vi "CRYStimulus.vi"(0 "Setup in":T2={"No.VI"=0, "Category"="", "StepName"="", "Seq setup flattened"="", "Comment"="", "Steps config."=[], "Jump config"=[], "Start"=0.0, "Increment"=0.0, "Name"="Pa", "Unit"="Pa", "Y data"=1, "Y prefix"="", "Y dB ref"=1.0, "Y unit"="", "Repeat State Array"=[]} {"Repeat State Array"."Start" format="%#_5g"; "Y dB ref" format="%.1f"; "Y data" items=["dB", "Lin"]; "Start" format="%#_5g"}, 5 "Data in":T10 {"Z data" items=["dB", "Lin"]; "X data" items=["dB", "Lin"]; "Y data" items=["dB", "Lin"]; "Z dB ref" format="%.1f"; "Z axis" items=["Log", "Lin"]; "X dB ref" format="%.1f"; "X axis" items=["Log", "Lin"]; "Y axis" items=["Log", "Lin"]; "Y dB ref" format="%.1f"; "Curve"."z" format="%.2f"; "Curve"."y" format="%.2f"; "Curve"."x" format="%.2f"}, 7 "Results in":T8 {"Margin" format="%.2f"}, 9 "Seq Setup in":string, 11 "Step name":string, 12 "Hardware in":string, 13 "Calibration in":string) -> (3 "Types Out":string[](array[string]), 4 "Inserted Names Out":string[](array[string]), 6 "Data out":T10 {"Z data" items=["dB", "Lin"]; "X data" items=["dB", "Lin"]; "Y data" items=["dB", "Lin"]; "Z dB ref" format="%.1f"; "Z axis" items=["Log", "Lin"]; "X dB ref" format="%.1f"; "X axis" items=["Log", "Lin"]; "Y axis" items=["Log", "Lin"]; "Y dB ref" format="%.1f"; "Curve"."z" format="%.2f"; "Curve"."y" format="%.2f"; "Curve"."x" format="%.2f"}, 8 "Results out":T8 {"Margin" format="%.2f"}, 10 "Wave out":T1[](array[typedef]) {"Y dB ref" format="%.1f"; "Y axis" items=["Log", "Lin"]; "Y data" items=["dB", "Lin"]; "X data" items=["dB", "Lin"]})   [LabVIEW 2013]
uses:
  Typedef Control/CRYData Cluster Array.ctl
  Typedef Control/CRYData Cluster.ctl
  Typedef Control/CRYResult Cluster Array.ctl
  Typedef Control/CRYResult Cluster.ctl
  Typedef Control/CRYWaveform Cluster.ctl
  Typedef Control/CRYCalibration 2DCluster.ctl
  Typedef Control/CRYCalibration Cluster.ctl
  Typedef Control/CRYStep.ctl
  Typedef Control/CRYStimulus Test Infor Cluster.ctl
  CRYMainGlobal.vi
  Task Sequence/CRYProject Run Control Global.vi
  Hardware/SubVI/CRY6175APT_Win32.dll
panel:
  out "Unit":u16
  out "Stop Amplitude":dbl
  in  "Start Amplitude":dbl
  in  "Frequency":dbl
  out "Steps":u32
  out "Resolution":u16
  in  "Stop Frequency":dbl
  in  "Start Frequency":dbl
  in  "Level Out":dbl
  in  "Sampling Rate":dbl
  in  "Sweep Time":dbl
  in  "Channel Out":i32=5
  out "use level":bool
  out "EQ Amplitude Rate":dbl
  out "Y dB ref":dbl
  in  "Waveform Cluster":T1={"Waveform"={"X0"=0.0, "dX"=0.0, "Y"=[]}, "X data"=1, "Y data"=0, "Y axis"=0, "X unit"="s", "Y unit"="", "Y dB ref"=1.0, "display Y"=TRUE, "display X"=FALSE, "Overload?"=FALSE, "Test Info"="", "Step No."=0, "Name"="", "protected"=FALSE, "Sqc history"=[], "Signal Channel ID"=0, "Plot Settings"={"Color"=0, "Interpolation"=0, "Point Style"=0, "Line Style"=0, "Point Color"=0, "Line Width"=0, "Bar Plot Style"=0, "Fill To"=0}, "AutoProtect"=FALSE} {"Y dB ref" format="%.1f"; "Y axis" items=["Log", "Lin"]; "Y data" items=["dB", "Lin"]; "X data" items=["dB", "Lin"]}
  out "EQ Curve":T3={"Name"="", "Curve"=[], "X data"=1, "Y data"=1, "Z data"=1, "X axis"=0, "Y axis"=1, "Z axis"=1, "X unit"="Hz", "Y unit"="", "Z unit"="deg.", "X dB ref"=1.0, "Y dB ref"=1.0, "Z dB ref"=1.0, "single val"=FALSE, "protected"=FALSE, "display X"=TRUE, "display Y"=TRUE, "display Z"=TRUE, "Test Info"="", "Step No."=0, "Plot Settings"={"Color"=0, "Interpolation"=0, "Point Style"=0, "Line Style"=0, "Point Color"=0, "Line Width"=0, "Bar Plot Style"=0, "Fill To"=0}, "AutoProtect"=FALSE} {"Z data" items=["dB", "Lin"]; "X data" items=["dB", "Lin"]; "Y data" items=["dB", "Lin"]; "Z dB ref" format="%.1f"; "Z axis" items=["Log", "Lin"]; "X dB ref" format="%.1f"; "X axis" items=["Log", "Lin"]; "Y axis" items=["Log", "Lin"]; "Y dB ref" format="%.1f"; "Curve"."z" format="%.2f"; "Curve"."y" format="%.2f"; "Curve"."x" format="%.2f"}
  out "Calibration All Cluster":T4={"Calibration"={"Calibration Step Name"="", "Device"="", "Correction Curve Name"="", "Equalization Curve Name"="", "Sensitivity Curve Name"="", "Corr Folder and File"="", "EQ Folder and File"="", "Sens Folder and File"="", "Corr Step size"=0, "EQ Step size"=0, "Input"=FALSE, "Last Cal Date (sec)"=timestamp(0 s since 1904-01-01), "Cha Name"="", "Corr Curve Found"=FALSE, "EQ Curve Found"=FALSE, "Sens Curve Found"=FALSE, "Signal Type"="", "Calibrated Device"="", "Hz"=0}, "Corr Curve"={"Name"="", "Curve"=[], "X data"=1, "Y data"=1, "Z data"=1, "X axis"=0, "Y axis"=1, "Z axis"=1, "X unit"="", "Y unit"="", "Z unit"="deg.", "X dB ref"=1.0, "Y dB ref"=1.0, "Z dB ref"=1.0, "single val"=FALSE, "protected"=FALSE, "display X"=FALSE, "display Y"=TRUE, "display Z"=TRUE, "Test Info"="", "Step No."=0, "Plot Settings"={"Color"=0, "Interpolation"=0, "Point Style"=0, "Line Style"=0, "Point Color"=0, "Line Width"=0, "Bar Plot Style"=0, "Fill To"=0}, "AutoProtect"=FALSE}, "EQ Curve"={"Name"="", "Curve"=[], "X data"=1, "Y data"=1, "Z data"=1, "X axis"=0, "Y axis"=1, "Z axis"=1, "X unit"="Hz", "Y unit"="", "Z unit"="deg.", "X dB ref"=1.0, "Y dB ref"=1.0, "Z dB ref"=1.0, "single val"=FALSE, "protected"=FALSE, "display X"=TRUE, "display Y"=TRUE, "display Z"=TRUE, "Test Info"="", "Step No."=0, "Plot Settings"={"Color"=0, "Interpolation"=0, "Point Style"=0, "Line Style"=0, "Point Color"=0, "Line Width"=0, "Bar Plot Style"=0, "Fill To"=0}, "AutoProtect"=FALSE}, "Sens Curve"={"Name"="", "Curve"=[], "X data"=1, "Y data"=1, "Z data"=1, "X axis"=0, "Y axis"=1, "Z axis"=1, "X unit"="Hz", "Y unit"="", "Z unit"="deg.", "X dB ref"=1.0, "Y dB ref"=1.0, "Z dB ref"=1.0, "single val"=FALSE, "protected"=FALSE, "display X"=TRUE, "display Y"=TRUE, "display Z"=TRUE, "Test Info"="", "Step No."=0, "Plot Settings"={"Color"=0, "Interpolation"=0, "Point Style"=0, "Line Style"=0, "Point Color"=0, "Line Width"=0, "Bar Plot Style"=0, "Fill To"=0}, "AutoProtect"=FALSE}} {"Sens Curve"."Z data" items=["dB", "Lin"]; "Sens Curve"."X data" items=["dB", "Lin"]; "Sens Curve"."Y data" items=["dB", "Lin"]; "Sens Curve"."Z dB ref" format="%.1f"; "Sens Curve"."Z axis" items=["Log", "Lin"]; "Sens Curve"."X dB ref" format="%.1f"; "Sens Curve"."X axis" items=["Log", "Lin"]; "Sens Curve"."Y axis" items=["Log", "Lin"]; "Sens Curve"."Y dB ref" format="%.1f"; "Sens Curve"."Curve"."z" format="%.2f"; "Sens Curve"."Curve"."y" format="%.2f"; "Sens Curve"."Curve"."x" format="%.2f"; "EQ Curve"."Z data" items=["dB", "Lin"]; "EQ Curve"."X data" items=["dB", "Lin"]; "EQ Curve"."Y data" items=["dB", "Lin"]; "EQ Curve"."Z dB ref" format="%.1f"; "EQ Curve"."Z axis" items=["Log", "Lin"]; "EQ Curve"."X dB ref" format="%.1f"; "EQ Curve"."X axis" items=["Log", "Lin"]; "EQ Curve"."Y axis" items=["Log", "Lin"]; "EQ Curve"."Y dB ref" format="%.1f"; "EQ Curve"."Curve"."z" format="%.2f"; "EQ Curve"."Curve"."y" format="%.2f"; "EQ Curve"."Curve"."x" format="%.2f"; "Corr Curve"."Z data" items=["dB", "Lin"]; "Corr Curve"."X data" items=["dB", "Lin"]; "Corr Curve"."Y data" items=["dB", "Lin"]; "Corr Curve"."Z dB ref" format="%.1f"; "Corr Curve"."Z axis" items=["Log", "Lin"]; "Corr Curve"."X dB ref" format="%.1f"; "Corr Curve"."X axis" items=["Log", "Lin"]; "Corr Curve"."Y axis" items=["Log", "Lin"]; "Corr Curve"."Y dB ref" format="%.1f"; "Corr Curve"."Curve"."z" format="%.2f"; "Corr Curve"."Curve"."y" format="%.2f"; "Corr Curve"."Curve"."x" format="%.2f"; "Calibration"."EQ Step size" items=["R10", "R20", "R40", "R80", "User"]; "Calibration"."Corr Step size" items=["R10", "R20", "R40", "R80", "User"]}
  out "Analysis Value":dbl[](array[numeric])
  out "TSR params":T6 {"Sweep Time" format="%.2f"; "Amplit" format="%.2f"; "FStop" format="%.2f"; "FStart" format="%.2f"; "FSamp" format="%.2f"; "Tsamp" format="%.2f"; "NHarm" format="%.2f"; "MStart" format="%.2f"; "MStop" format="%.2f"; "NOffset" format="%.2f"}
  out "FAPS":T7(array[cluster]) {"cycles" format="%.2f"; "ampl" format="%.2f"; "freq" format="%.2f"}
  in  "Channel In":i32
  in  "wav path":path
  in  "max level":dbl format="%.2f"
  in  "Eq":cluster{"Hz":sgl, "dB":sgl, "Deg":sgl}[](array[cluster]) {"Deg" format="%.1f"; "dB" format="%.1f"}
  out "EQ Step size":u16(ring)=4 items=["R10", "R20", "R40", "R80", "User"]
  out "EQ Steps":i32=19
  in  "sine waves":cluster{"freq":dbl, "ampl":dbl, "cycles":dbl}[](array[cluster]) {"cycles" format="%.2f"; "ampl" format="%.2f"; "freq" format="%.2f"}
  in  "sweep type":i32
  out "Y unit":string
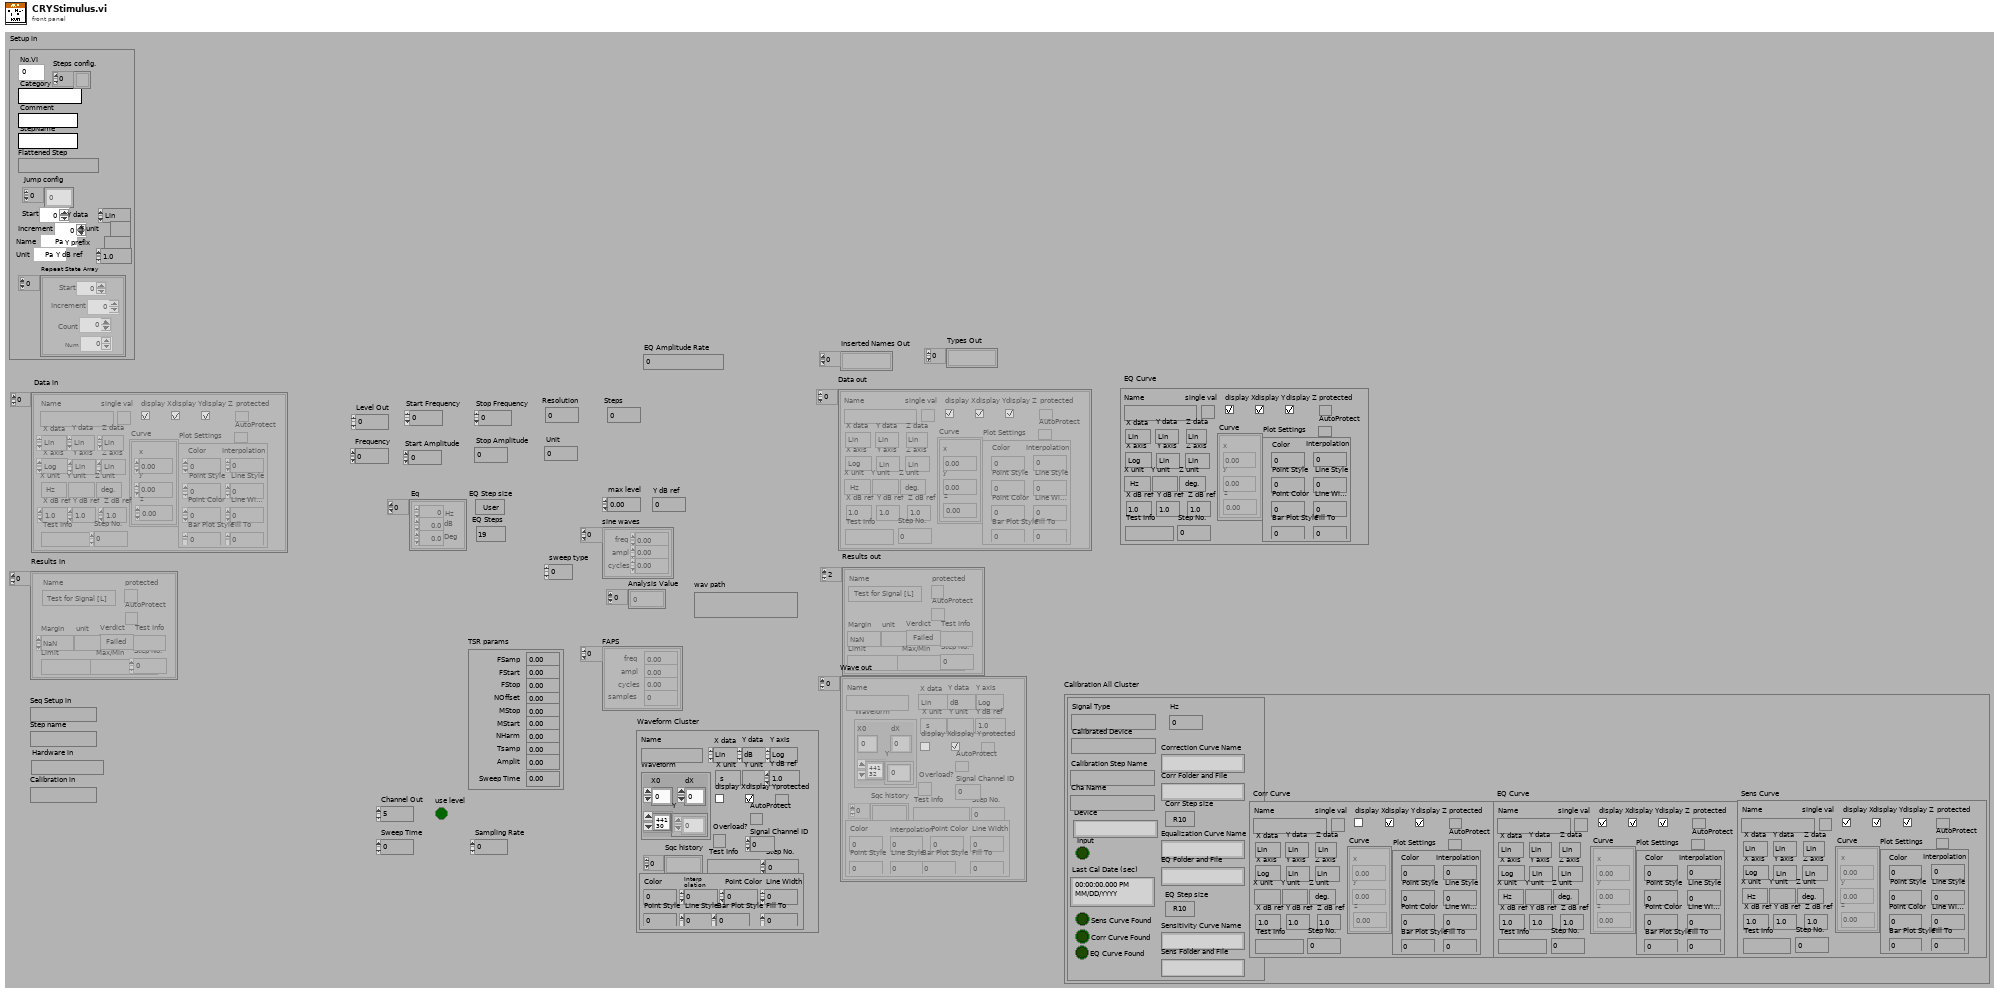
[diagram p1: front panel]
types:
  T1 = typedef "CRYWaveform Cluster.ctl" = cluster{"Waveform":cluster{"X0":dbl, "dX":dbl, "Y":sgl[]}, "X data":u16, "Y data":u16, "Y axis":u16, "X unit":string, "Y unit":string, "Y dB ref":dbl, "display Y":bool, "display X":bool, "Overload?":bool, "Test Info":string, "Step No.":i32, "Name":string, "protected":bool, "Sqc history":string[], "Signal Channel ID":i32, "Plot Settings":cluster{"Color":u32, "Interpolation":u8, "Point Style":u8, "Line Style":u8, "Point Color":u32, "Line Width":u8, "Bar Plot Style":u8, "Fill To":i16}, "AutoProtect":bool}
  T2 = typedef "CRYStep.ctl" = cluster{"No.VI":i32, "Category":string, "StepName":string, "Seq setup flattened":string, "Comment":string, "Steps config.":bool[], "Jump config":i32[], "Start":dbl, "Increment":dbl, "Name":string, "Unit":string, "Y data":u16, "Y prefix":string, "Y dB ref":dbl, "Y unit":string, "Repeat State Array":cluster{"Start":dbl, "Increment":dbl, "Count":i32, "Num":i32}[]}
  T3 = typedef "CRYData Cluster.ctl" = cluster{"Name":string, "Curve":cluster{"x":dbl, "y":dbl, "z":dbl}[], "X data":u16, "Y data":u16, "Z data":u16, "X axis":u16, "Y axis":u16, "Z axis":u16, "X unit":string, "Y unit":string, "Z unit":string, "X dB ref":dbl, "Y dB ref":dbl, "Z dB ref":dbl, "single val":bool, "protected":bool, "display X":bool, "display Y":bool, "display Z":bool, "Test Info":string, "Step No.":i32, "Plot Settings":cluster{"Color":u32, "Interpolation":u8, "Point Style":u8, "Line Style":u8, "Point Color":u32, "Line Width":u8, "Bar Plot Style":u8, "Fill To":i16}, "AutoProtect":bool}
  T4 = typedef "CRYCalibration 2DCluster.ctl" = cluster{"Calibration":T5, "Corr Curve":T3, "EQ Curve":T3, "Sens Curve":T3}
  T5 = typedef "CRYCalibration Cluster.ctl" = cluster{"Calibration Step Name":string, "Device":string, "Correction Curve Name":string, "Equalization Curve Name":string, "Sensitivity Curve Name":string, "Corr Folder and File":string, "EQ Folder and File":string, "Sens Folder and File":string, "Corr Step size":u16, "EQ Step size":u16, "Input":bool, "Last Cal Date (sec)":timestamp, "Cha Name":string, "Corr Curve Found":bool, "EQ Curve Found":bool, "Sens Curve Found":bool, "Signal Type":string, "Calibrated Device":string, "Hz":u32}
  T6 = cluster{"FSamp":dbl, "FStart":dbl, "FStop":dbl, "NOffset":dbl, "MStop":dbl, "MStart":dbl, "NHarm":dbl, "Tsamp":dbl, "Amplit":dbl, "Sweep Time":dbl}
  T7 = cluster{"freq":dbl, "ampl":dbl, "cycles":dbl, "samples":i32}[]
  T8 = typedef "CRYResult Cluster Array.ctl" = T9[]
  T9 = typedef "CRYResult Cluster.ctl" = cluster{"Name":string, "Margin":dbl, "unit":string, "Verdict":bool, "Limit":string, "Max/Min":string, "protected":bool, "Step No.":i32, "Test Info":string, "AutoProtect":bool}
  T10 = typedef "CRYData Cluster Array.ctl" = T3[]
  T11 = enum16{"OK", "Yes", "YesNo", "YesNoCancel", "ReplaceAppend"}
  T12 = cluster{"FSamp":dbl, "FStart":dbl, "FStop":dbl, "NOffset":dbl, "MStop":dbl, "MStart":dbl, "NHarm":dbl, "Tsamp":dbl, "Amplit":dbl, "Amplit 2":dbl}
  T13 = cluster{"Start":dbl, "Increment":dbl, "Count":i32, "Num":i32}[]
  T14 = typedef "CRYStimulus Cluster.ctl" = cluster{"StimulusType":string, "UseMLValArray":u16[], "ML_axisArray":u16[], "MLValLevelNameArray":string[], "Level(U)Array":dbl[], "Start(Stop)FreqArray":dbl[], "Start(Stop)AmpArray":dbl[], "StepResolutionArray":u16[], "Unit_Array":u16[], "DegValArray":dbl[], "DegUnitArray":string[], "Steps1":i32, "Cycle/step1(#)":u32, "Time/step1(s)":dbl, "Transition1":dbl, "SweepRate2":dbl, "Freq3(Hz)":dbl, "Steps3(#)":dbl, "Cycles3(#)":u32, "StepSize3":dbl, "wave time":string, "RMS_Value4":dbl, "Peak_Value4":dbl, "WavePath4":string, "RMS_unit4":string, "Peak_unit4":string, "wave Info":string, "dc_ctrl5_1":u16, "dc_ctrl5_2":u16, "dc_polar5":u16, "Max.Current":u16, "Steps5(#)":u32, "Time/Step5":dbl, "Level5":dbl, "StepsSize5Val":dbl, "StepSize5Unit":string, "SweepType":u16, "Fixed/Ratio6":u16, "Transition6":dbl, "Steps6(#)":dbl, "Cycle/Steps6(#)":u32, "Time/Steps6(s)":dbl, "Freq6(Hz)":dbl, "Difference6(Hz)":dbl, "Ratio6":string, "NoiseType7":u16, "Duration7(s)":dbl, "MinFreq7(Hz)":dbl, "MaxFreq7(Hz)":dbl, "MinFreq8(Hz)":dbl, "MaxFreq8(Hz)":dbl, "FreqRounding8":bool, "Duration8(s)":dbl, "Tones8":dbl, "RoundingVal8":dbl, "ApplyEQ":bool, "Duration(s)":dbl, "CustomStimulusName ":string, "Flatten Element Array":string[], "sine waves":cluster{"freq":dbl, "ampl":dbl, "cycles":dbl}[], "Channel Out":i32, "RatioVal6":dbl, "TabCtrl6":enum32{"Master Tone", "Slave Tone"}, "Signal Type Name":string, "Help":string, "Channel Sel":u16, "V on DUT":bool, "Output Imp":dbl, "Nominal Imp":dbl}
  T15 = typedef "CRYStimulus Parameter.ctl" = cluster{"Name":string, "Level Out":dbl, "Start Freq":dbl, "Stop Freq":dbl, "Steps":u32, "Cycles":u32, "Sweep type":i32, "Freq":dbl, "Start ampl":dbl, "Stop ampl":dbl, "sine waves":cluster{"freq":dbl, "ampl":dbl, "cycles":dbl}[], "wav path":string, "Sweep time":dbl, "Resolution":u16, "Tone type6":u16, "fix/ratio6":u16, "Ratio6":u16, "Difference6":u32, "RatioFreq6":u32}
  T16 = typedef "CRYfstepsw.ctl" = cluster{"Level(U)":dbl, "Start Freq(Hz)":dbl, "Stop Freq(Hz)":dbl, "ML val level name":string, "Use ML Val level?":bool, "ML axis":u8, "Steps (#)":i32, "Cycles/step(#)":u32, "Time/step (s)":dbl, "Step Resolution":u16, "unit":u16, "Start Freq Name":string, "Stop Freq Name":string, "Start Freq Axis":u8, "Stop Freq Axis":u8, "Start Freq Flag":string, "Stop Freq Flag":string, "Output Imp":dbl, "Nominal Imp":dbl, "V on DUT":bool}
  T17 = typedef "CRYflogsw.ctl" = cluster{"Level(U)":dbl, "Start Freq(Hz)":dbl, "Stop Freq(Hz)":dbl, "Sweep Rate(s/dec)":dbl, "Use ML Val level?":bool, "ML val level name":string, "ML axis":u8, "TSR params":cluster{"FSamp":dbl, "FStart":dbl, "FStop":dbl, "NOffset":dbl, "MStop":dbl, "MStart":dbl, "NHarm":dbl, "Tsamp":dbl, "Amplit":dbl}, "unit":u16, "Start Freq Name":string, "Stop Freq Name":string, "Start Freq Axis":u8, "Stop Freq Axis":u8, "Start Freq Flag":string, "Stop Freq Flag":string, "Output Imp":dbl, "Nominal Imp":dbl, "V on DUT":bool}
  T18 = typedef "CRYampsw.ctl" = cluster{"Freq(Hz)":dbl, "Steps (#)":i32, "Cycles(#)":u32, "Use ML Val freq?":bool, "ML val freq name":string, "ML axis":u8, "Start Ampl(U)":dbl, "Stop Ampl(U)":dbl, "unit":u16}
  T19 = typedef "CRYwavefile.ctl" = cluster{"Level(U)":dbl, "Wave Path":string, "ML axis":u8, "ML val level name":string, "Use ML Val level?":bool, "wave info":string, "wave time":string, "Peak value4":dbl, "RMS value4":dbl, "wave channel":u16, "unit":u16, "Output Imp":dbl, "Nominal Imp":dbl, "V on DUT":bool}
  T20 = typedef "CRYdcconn.ctl" = cluster{"dc ctrl":u16, "dcmax I":u16, "dc polar":u16, "dc ctrl":u16, "Steps (#)":i32, "Time/step (s)":dbl, "Start Ampl(U)":dbl, "Stop Ampl(U)":dbl, "Level(U)":dbl, "Step Size":dbl}
  T21 = typedef "CRYtwotone.ctl" = cluster{"Steps (#)":i32, "Tone Type":u8, "Freq2(Hz)":dbl, "Time/step (s)":dbl, "Cycles/step (#)":u32, "ML val level name":string, "Use ML Val level?":bool, "Level(U) 2":dbl, "Diff Freq(Hz)":dbl, "ML axis 2":u8, "Diff/Ratio":u8, "Level(U)":dbl, "Stop Freq(Hz)":dbl, "Ratio Val":dbl, "ML val level name 2":string, "Use ML Val level? 2":bool, "ML axis":u8, "Start Freq(Hz)":dbl, "Step Resolution":u16, "Ratio":u16, "TabCtrl6":enum32{"Master Tone", "Slave Tone"}, "unit 1":u16, "unit 2":u16, "Start Freq Name":string, "Stop Freq Name":string, "Start Freq Axis":u8, "Stop Freq Axis":u8, "Start Freq Flag":string, "Stop Freq Flag":string}
  T22 = typedef "CRYmltitone.ctl" = cluster{"Level(U)":dbl, "Min Freq(Hz)":dbl, "Max Freq(Hz)":dbl, "Duration(s)":dbl, "Freq Rounding":bool, "Rounding Val":dbl, "Profile":i32, "ML axis 2":u8, "ML val level name":string, "Use ML Val level?":bool, "ML axis":u8, "Step Resolution":u16, "unit":u16, "Start Freq Name":string, "Stop Freq Name":string, "Start Freq Axis":u8, "Stop Freq Axis":u8, "Start Freq Flag":string, "Stop Freq Flag":string, "Output Imp":dbl, "Nominal Imp":dbl, "V on DUT":bool}
  T23 = typedef "CRYnoise.ctl" = cluster{"Noise Type":u8, "Min Freq(Hz)":dbl, "Max Freq(Hz)":dbl, "Level(U)":dbl, "Duration(s)":dbl, "ML val level name":string, "Use ML Val level?":bool, "ML axis":u8, "unit":u16, "Start Freq Name":string, "Stop Freq Name":string, "Start Freq Axis":u8, "Stop Freq Axis":u8, "Start Freq Flag":string, "Stop Freq Flag":string, "Output Imp":dbl, "Nominal Imp":dbl, "V on DUT":bool}
  T24 = cluster{"fstepsw":T16, "flogsw":T17, "ampsw":T18, "wavefile":T19, "dcconn":T20, "twotone":T21, "mltitone":T22, "noise":T23, "sqwvsw":cluster{"Level(U)":dbl, "Duty Cycle":dbl, "ML val level name":string, "ML axis":u8, "Start Freq(Hz)":u32, "Stop Freq(Hz)":u32, "Use ML Val level?":bool, "Steps (#)":u32, "Cycles/step (#)":u32, "Time/step (s)":dbl, "Step Resolution":u16}, "tnbrst":cluster{"Level(U)":dbl, "ML val level name":string, "ML axis":u8, "Start Freq(Hz)":u32, "Use ML Val level?":bool, "Cycles/step (#)":u32, "Duration(s)":dbl}}
  T25 = typedef "CRYHardware Channel Info.ctl" = cluster{"ID":i32, "Name":string, "Digital":bool, "Input":bool, "Device Name":string, "Hardware Ch ID":u8, "Vmax (V)":dbl, "Latency (samples)":dbl, "Sampling Rate (Hz)":u32, "Bit Depth":u32, "Anti-aliasing Factor (%fs)":sgl, "DAQmx Channel":tag, "term config":i32, "Coupling":i32, "IEPE en":bool, "ASIOChannel Name":string, "Audio Driver":u16, "ASIOChannel Index":u8}
  T26 = cluster{"sweep type":i32, "Sampling Rate":dbl, "Frequency":dbl, "Start Amplitude":dbl, "Level Out":dbl}
  T27 = cluster{"Unit":u16, "max level":dbl, "Y dB ref":dbl}
  T28 = cluster{"Start Frequency":dbl, "Stop Frequency":dbl, "Steps":u32, "Sweep Time":dbl, "Level Out":dbl, "Level Out":dbl, "Unit":u16, "max level":dbl, "Y dB ref":dbl}
  T29 = typedef "CRYStimulus Test Infor Cluster.ctl" = cluster{"Stimulus Type":string, "Signal Type":string, "In/Out":bool, "FAPS":cluster{"freq":dbl, "ampl":dbl, "cycles":dbl, "samples":i32}[], "Sampling Rate":dbl, "Samples":i32, "Analysis Param":string, "Resolution":u16, "Steps":u32, "Analysis Value":dbl[], "Diff Freq":dbl, "FStart":dbl, "FStop":dbl, "Calibration Param":string, "Anti Alias":dbl, "Level Out1":dbl, "Level Out2":dbl, "EQ":bool}
  T30 = typedef "CRYWaveform Cluster Array.ctl" = T1[]
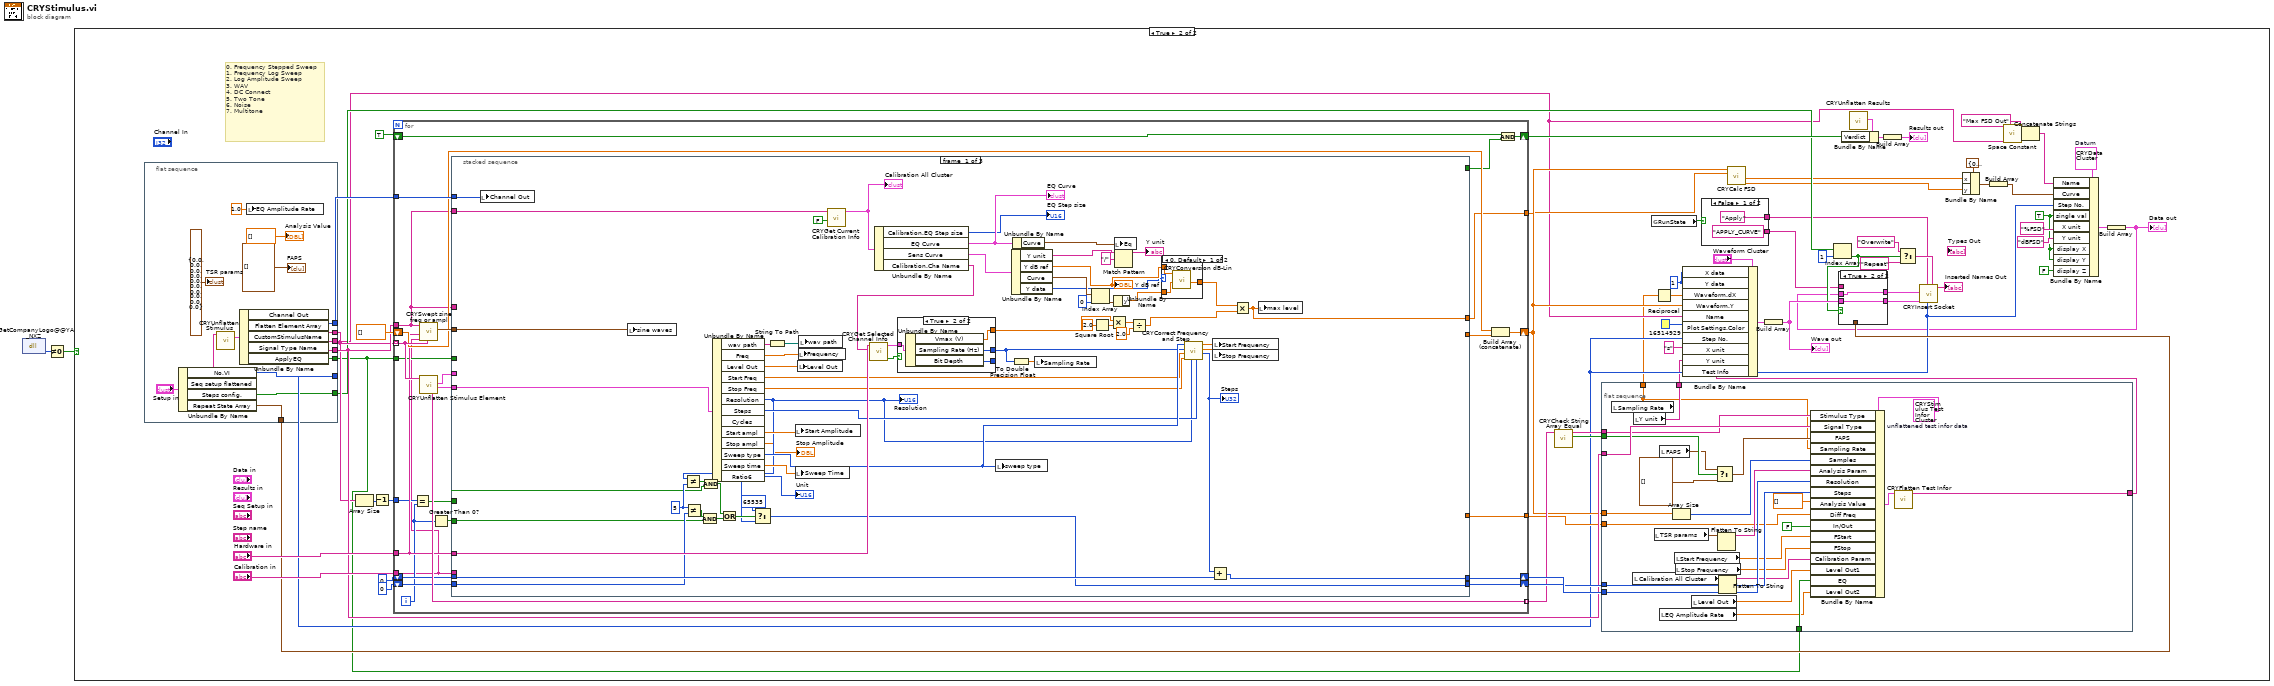
[diagram p0: block diagram]
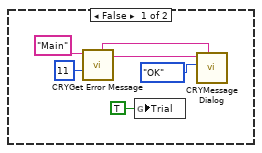
[diagram p2: hidden frame]
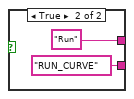
[diagram p3: hidden frame]
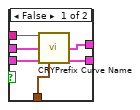
[diagram p4: hidden frame]
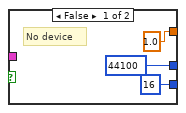
[diagram p6: hidden frame]
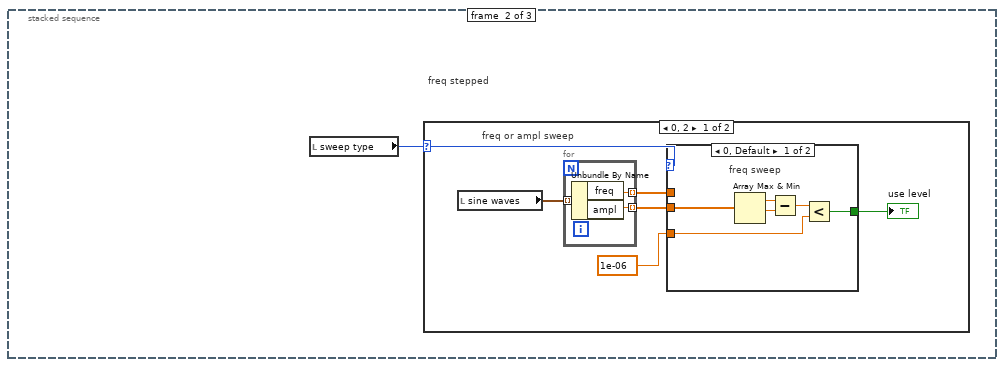
[diagram p7: hidden frame]
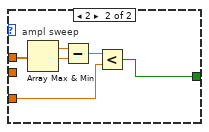
[diagram p8: hidden frame]
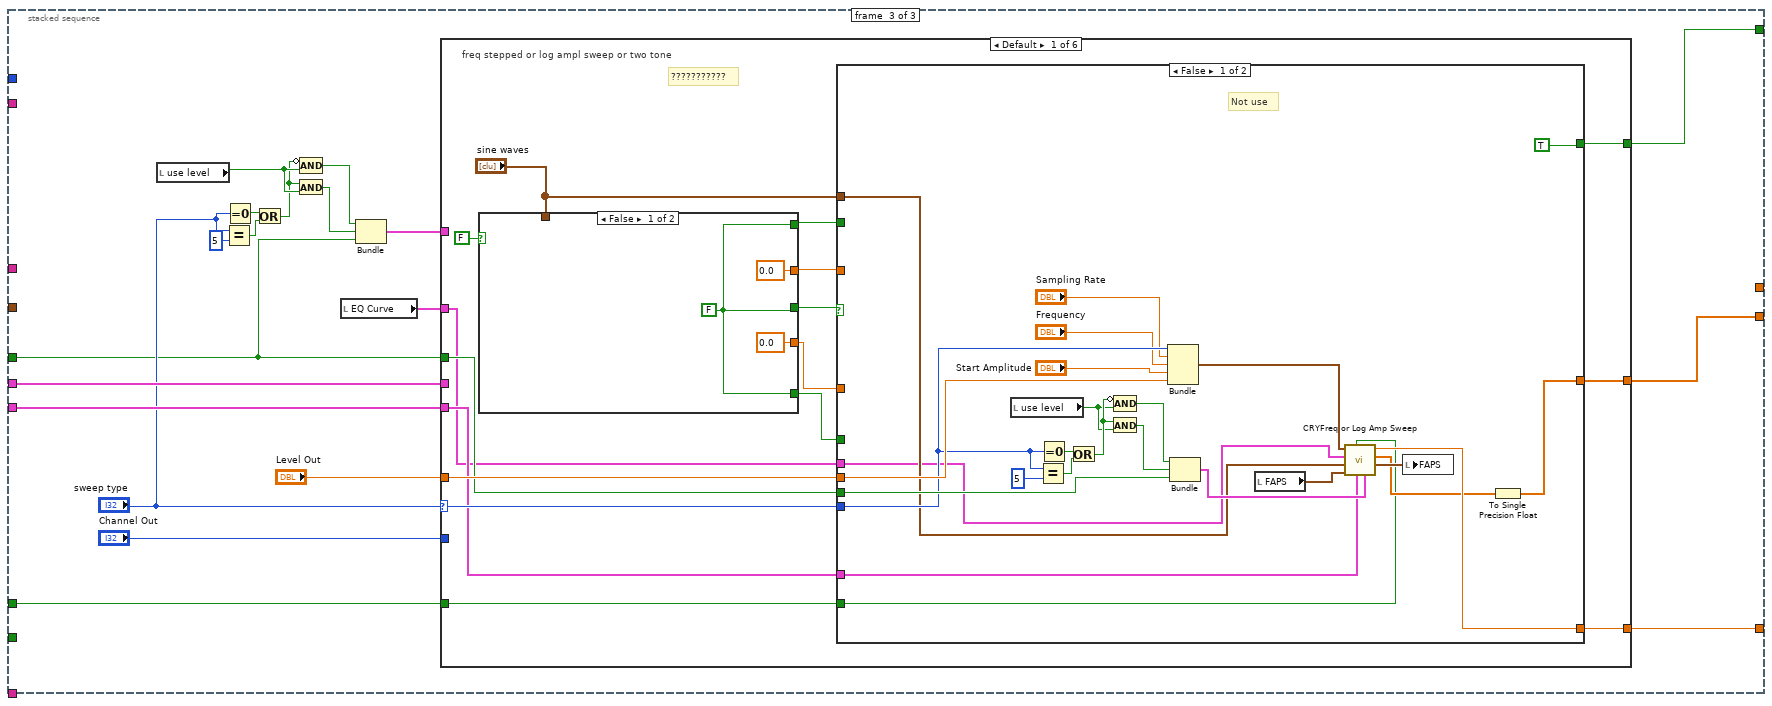
[diagram p10: hidden frame]
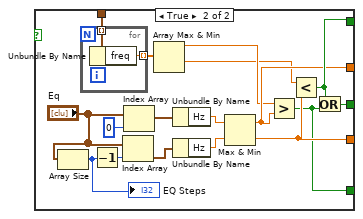
[diagram p11: hidden frame]
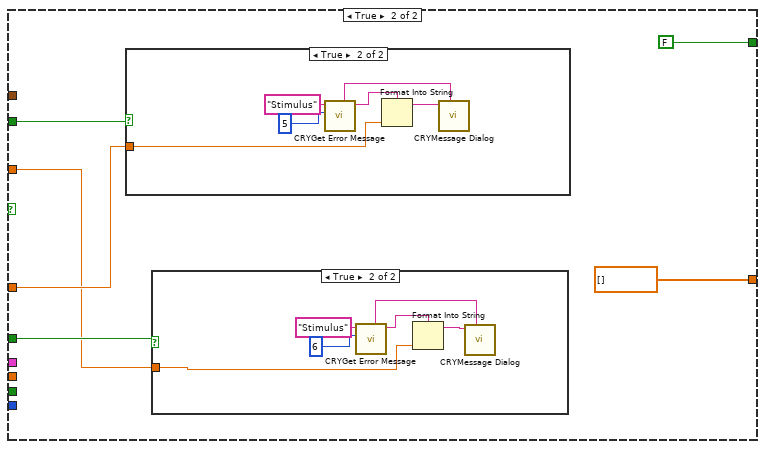
[diagram p12: hidden frame]
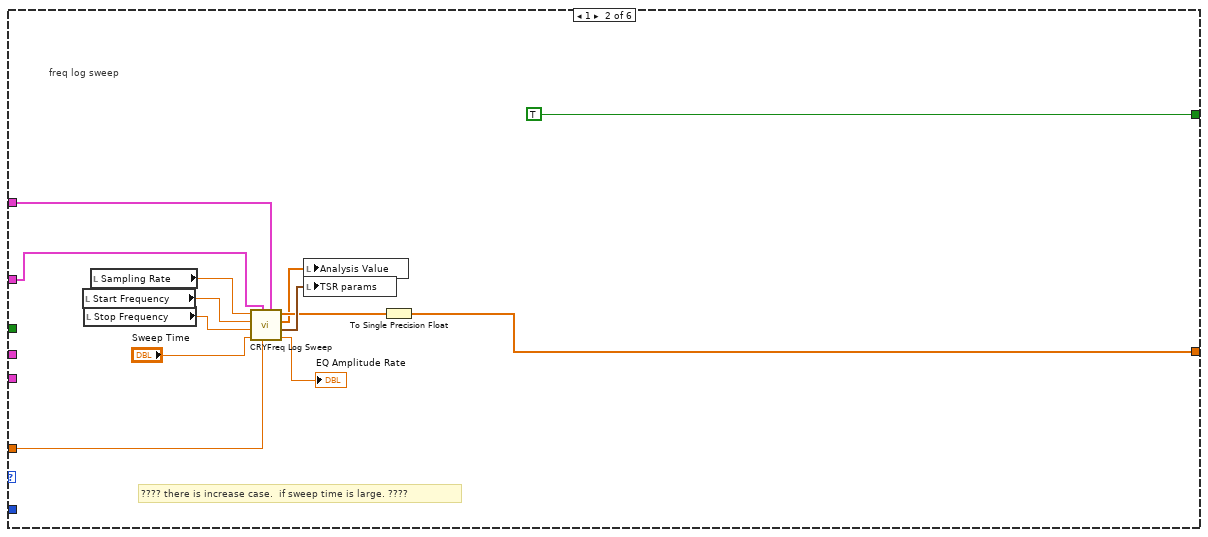
[diagram p15: hidden frame]
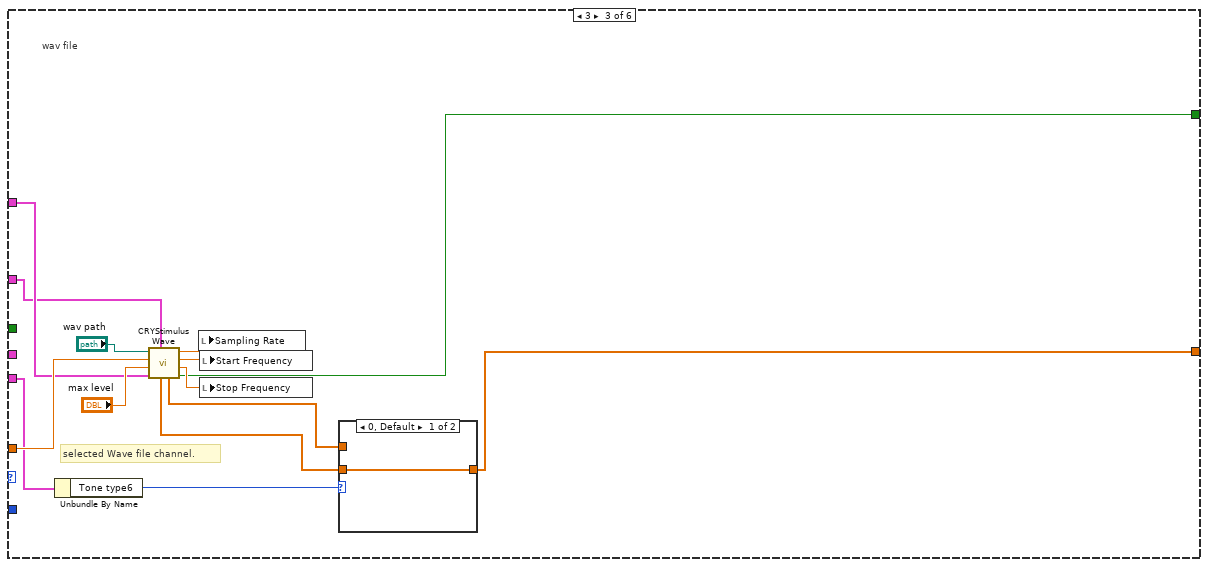
[diagram p16: hidden frame]
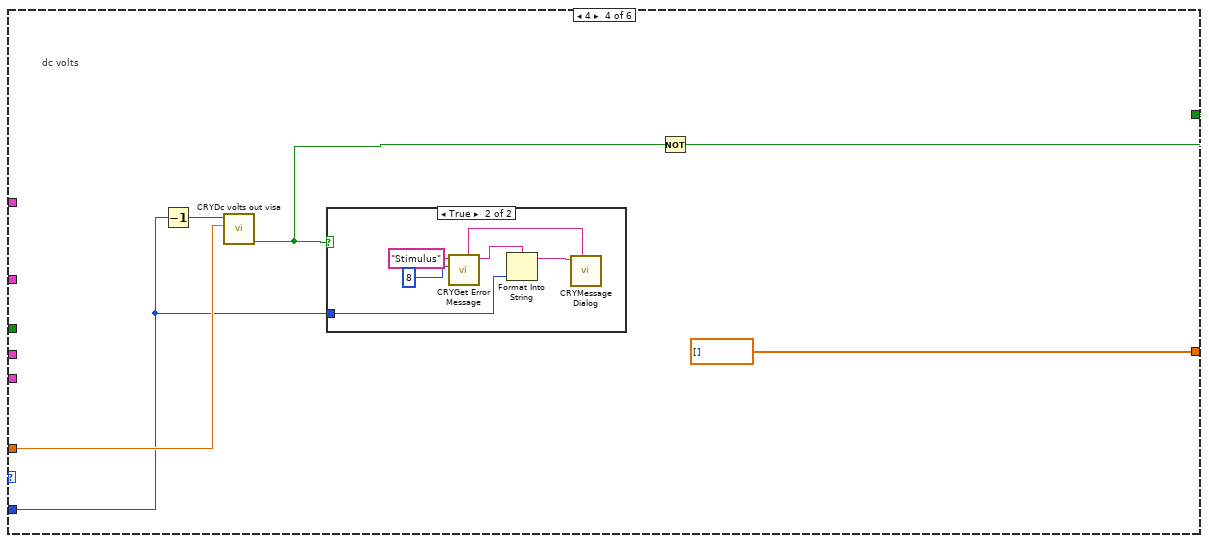
[diagram p18: hidden frame]
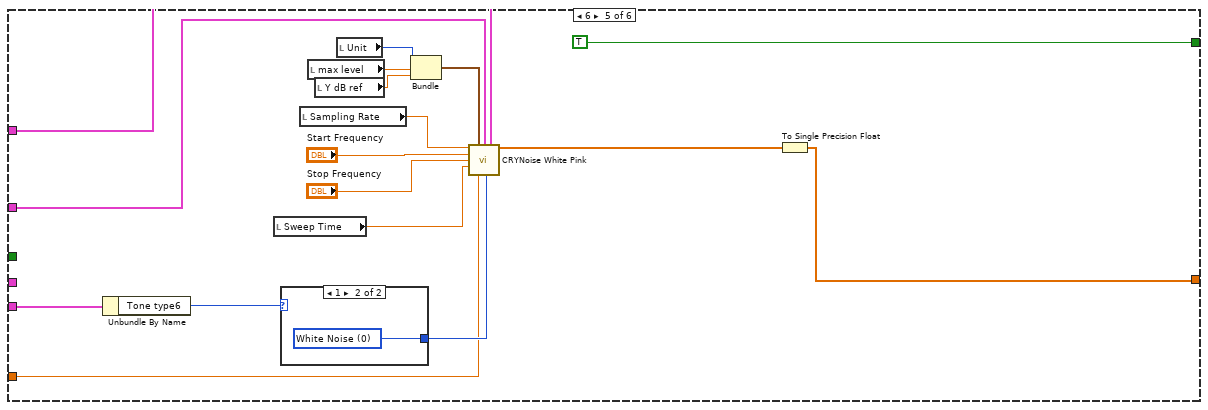
[diagram p20: hidden frame]
diagram:
  n1 = dll-call lib="D:/A_CRYSoundLab_Work/CRY6181/CRYSystem/Hardware/SubVI/CRY6175APT_Win32.dll" fn="?GetCompanyLogo@@YA_NXZ"() -> ("return type"=w2:i32)  [unwired: 3 in, 2 out]
  n2 = Not Equal To 0?(x=w2) -> (x != 0?=w1:bool)
  n3 = case shown="True" w1 {
    frame False {
      n4 = call "CRYGet Error Message.vi"("Error No"=11, "Kind"="Main") -> ("Message"=w3:string, "Window Title"=w7:string)  [unwired: 4 in, 4 out]
      n5 = global write "CRYMainGlobal.vi" "Trial"(TRUE ("Trial")) -> ()
      n6 = call "CRYMessage Dialog.vi"("Window Title"=w7, "YesNoCancel"=T11."OK", "Message Content"=w3) -> ()  [unwired: 7 in, 2 out]
    }
    frame True {
      w30 = T3 {"Name"="", "Curve"=[], "X data"=1, "Y data"=1, "Z data"=1, "X axis"=0, "Y axis"=1, "Z axis"=1, "X unit"="Hz", "Y unit"="", "Z unit"="deg.", "X dB ref"=1.0, "Y dB ref"=1.0, "Z dB ref"=1.0, "single val"=FALSE, "protected"=FALSE, "display X"=TRUE, "display Y"=TRUE, "display Z"=FALSE, "Test Info"="", "Step No."=0, "Plot Settings"={"Color"=0, "Interpolation"=0, "Point Style"=0, "Line Style"=0, "Point Color"=0, "Line Width"=0, "Bar Plot Style"=0, "Fill To"=0}, "AutoProtect"=FALSE}  # Datum
      w10 = TRUE ("single val")
      w46 = u16 1 ("X data")
      # "0. Frequency Stepped Sweep\n1. Frequency Log Sweep\n2. Log Amplitude Sweep\n3. WAV\n4. DC Connect\n5. Two Tone\n6. Noise\n7. Multitone"
      n7 = flat-sequence {
        tunnel: [w125] -> w64
        tunnel: [w118] -> w58
        tunnel: [w119] -> w15
        tunnel: [w124] -> w59
        tunnel: [w121] -> w9
        tunnel: [w115] -> w26
        tunnel: [w114] -> w55
        tunnel: [w113] -> w54
        frame #0 {
          n8 = Unbundle By Name("Setup in") -> ("No.VI"=w115:i32, "Seq setup flattened"=w116:string, "Steps config."=w114:bool[], "Repeat State Array"=w113:T13)
          n9 = call "CRYUnflatten Stimulus.vi"("Flatten Stimulus"=w116) -> ("Stimulus"=w126:T14)  [unwired: 10 out]
          n10 = Unbundle By Name(w126) -> ("Channel Out"=w125:i32, "Flatten Element Array"=w118:string[], "CustomStimulusName"=w119:string, "Signal Type Name"=w124:string, "ApplyEQ"=w121:bool)
          n11 = local write "EQ Amplitude Rate"(1.0 ("EQ Amplitude Rate")) -> ()
          "FAPS" <- T7 [] ("FAPS")
          "TSR params" <- T12 {"FSamp"=0.0, "FStart"=0.0, "FStop"=0.0, "NOffset"=0.0, "MStop"=0.0, "MStart"=0.0, "NHarm"=0.0, "Tsamp"=0.0, "Amplit"=0.0, "Amplit 2"=0.0} ("TSR params")
          "Analysis Value" <- dbl[] [] ("Analysis Value")
        }
      }
      n12 = Array Size(array=w58) -> (size(s)=w57:i32)
      n13 = Decrement(x=w57) -> (x-1=w56:i32)
      n14 = for {
        tunnel: w64 -> [w152]
        tunnel: "Hardware in" -> [w136]
        tunnel: "Calibration in" -> [w127]
        tunnel: w58 -> [w150] mode=indexing
        shift-right: [w147] -> w31
        shift-left: sgl[] [] ("Stimulus time points") -> [w148]
        shift-right: [w145] -> w66
        shift-left: TRUE ("Verdict") -> [w143]
        tunnel: [w142] -> w53 mode=indexing
        shift-right: [w140] -> w63
        shift-left: u16 0 ("Resolution") -> [w137]
        shift-right: [w139] -> w60
        shift-left: u32 0 ("Steps") -> [w138]
        tunnel: w59 -> [w129]
        tunnel: w9 -> [w135]
        tunnel: [w134] -> w32
        tunnel: w56 -> [w132]
        tunnel: [w128] -> w18
        i -> [w131]
        n15 = Equal?(x=w132, y=w131) -> (x = y?=w130:bool)
        n16 = call "CRYSwept sine freq or ampl.vi"("Stimulus setup"=w150, "Calibration setup"=w127, "Hardware setup"=w136, "Signal Path"=w129) -> ("Master"=w151:cluster{"freq":dbl, "ampl":dbl, "cycles":dbl}[])  [unwired: 7 out]
        n17 = call "CRYUnflatten Stimulus Element.vi"("Unflatten Stimulus Element setup"=w150) -> ("Stimulus Para"=w149:T15, "Stimulus Default"=w133:T24, "Type Name"=w142:string)  [unwired: 1 in, 7 out]
        n18 = Greater Than 0?(x=w131) -> (x > 0?=w141:bool)
        n19 = stacked-sequence {
          tunnel: w152 -> [w206 _ _]
          tunnel: w136 -> [w202 _ _]
          tunnel: w127 -> [_ _ _]
          tunnel: w149 -> [w204 _ w264]
          tunnel: w151 -> [w203 _ _]
          tunnel: [_ _ w260] -> w146
          tunnel: [_ _ w265] -> w144
          tunnel: w141 -> [w194 _ _]
          tunnel: [w199 _ _] -> w140
          tunnel: [w200 _ _] -> w139
          tunnel: w138 -> [w201 _ _]
          tunnel: w137 -> [w197 _ _]
          tunnel: w129 -> [w179 _ _]
          tunnel: w135 -> [_ _ w251]
          tunnel: [_ _ w263] -> w134
          tunnel: w133 -> [_ _ w262]
          tunnel: w130 -> [_ _ w261]
          tunnel: w129 -> [_ _ _]
          tunnel: [w158 _ _] -> w128
          frame #0 {
            w195 = u16 5 ("y")
            n20 = local write "Channel Out"(w206) -> ()
            n21 = local write "sine waves"(w203) -> ()
            n22 = Not Equal?(x=w195, y=w197) -> (x != y?=w196:bool)
            n23 = Compound Arithmetic op=AND(w196, w194) -> (w191:bool)
            n24 = Unbundle By Name(w204) -> ("wav path"=w207:string, "Freq"=w208:dbl, "Level Out"=w209:dbl, "Start Freq"=w185:dbl, "Stop Freq"=w184:dbl, "Resolution"=w156:u16, "Steps"=w183:u32, "Start ampl"=w211:dbl, "Stop ampl"=→"Stop Amplitude":dbl, "Sweep type"=w189:i32, "Sweep time"=w205:dbl, "Ratio6"=→"Unit":u16)  [unwired: 1 out]
            "Resolution" <- w156
            n25 = Not Equal?(x=w156, y=w195) -> (x != y?=w193:bool)
            n26 = Compound Arithmetic op=AND(w193, w194) -> (w192:bool)
            n27 = Or(x=w192, y=w191) -> (x .or. y?=w190:bool)
            n28 = Select(t=u16 65535, s=w190, f=w156) -> (s? t:f=w199:u16)
            n29 = String To Path(string=w207) -> (path=w210:path)
            n30 = local write "Start Amplitude"(w211) -> ()
            n31 = local write "Sweep Time"(w205) -> ()
            n32 = local write "Level Out"(w209) -> ()
            n33 = local write "Frequency"(w208) -> ()
            n34 = local write "wav path"(w210) -> ()
            n35 = call "CRYGet Current Calibration Info.vi"("Is Input?"=FALSE, "Signal Type Name"=w179) -> ("Calibration All Cluster"=w177:T4)  [unwired: 9 out]
            "Calibration All Cluster" <- w177
            n36 = Unbundle By Name(w177) -> ("Calibration.EQ Step size"=→"EQ Step size":u16, "EQ Curve"=w181:T3, "Sens Curve"=w180:T3, "Calibration.Cha Name"=w169:string)
            "EQ Curve" <- w181
            n37 = call "CRYGet Selected Channel Info.vi"("Channel Name"=w169, "Flattened Hardware"=w202) -> ("exist?"=w171:bool, "Channel infor"=w172:T25)  [unwired: 1 in, 7 out]
            n38 = case shown="True" w171 {
              tunnel: [u32 44100 ("Sampling Rate (Hz)") w224] -> w186
              tunnel: [1.0 ("Vmax (V)") w223] -> w166
              tunnel: w172 -> [_ w222]
              tunnel: [u32 16 ("Bit Depth") w221] -> _
              frame False {
                # "No device"
              }
              frame True {
                n39 = Unbundle By Name(w222) -> ("Vmax (V)"=w223:dbl, "Sampling Rate (Hz)"=w224:u32, "Bit Depth"=w221:u32)
              }
            }
            n40 = local write "sweep type"(w189) -> ()
            n41 = Unbundle By Name(w180) -> ("Y unit"=w157:string, "Y dB ref"=w164:dbl, "Curve"=w174:cluster{"x":dbl, "y":dbl, "z":dbl}[], "Y data"=w162:u16)
            "Y dB ref" <- w164
            n42 = Unbundle By Name(w181) -> ("Curve"=w178:cluster{"x":dbl, "y":dbl, "z":dbl}[])
            n43 = To Double Precision Float(number=w186) -> (double precision float=w170:dbl)
            n44 = local write "Sampling Rate"(w170) -> ()
            n45 = Index Array(array=w174, index=0) -> (element=w173:cluster{"x":dbl, "y":dbl, "z":dbl})
            n46 = Square Root(x=2.0) -> (sqrt(x)=w161:dbl)
            n47 = Multiply(x=w166, y=w161) -> (x*y=w160:dbl)
            n48 = Unbundle By Name(w173) -> ("y"=w163:dbl)
            n49 = local write "Eq"(w178) -> ()
            n50 = Match Pattern(string=w157, regular expression="/") -> (before substring=→"Y unit":string)  [unwired: 4 out]
            n51 = Divide(x=w160, y=2.0) -> (x/y=w165:dbl)
            n52 = case shown="0, Default" w162 {
              tunnel: w163 -> [w216 w217]
              tunnel: [w215 w217] -> w159
              tunnel: w164 -> [w214 _]
              frame 0, Default {
                n53 = call "CRYConversion dB-Lin.vi"("dB ref."=w214, "Log In"=w216) -> ("Lin Out"=w215:dbl)  [unwired: 4 in, 3 out]
              }
              frame 1 {
              }
            }
            n54 = call "CRYCorrect Frequency and Step.vi"("Steps"=w183, "Resolution"=w156, "Stop Frequency"=w184, "Start Frequency"=w185, "Sampling Rate"=w186, "Sweep type"=w189) -> ("Steps"=w155:u32, "Stop Freq Out"=w187:dbl, "Start Freq Out"=w188:dbl)  [unwired: 3 in]
            "Steps" <- w155
            n55 = Add(x=w155, y=w201) -> (x+y=w200:u32)
            n56 = local write "Start Frequency"(w188) -> ()
            n57 = local write "Stop Frequency"(w187) -> ()
            n58 = Multiply(x=w159, y=w165) -> (x*y=w158:dbl)
            n59 = local write "max level"(w158) -> ()
          }
          frame #1 {
            # "freq stepped"
            n60 = local read "sweep type"() -> (w225:i32)
            n61 = case shown="0, 2" w225 {
              selector: w225 -> [w226 _]
              frame 0, 2 {
                # "freq or ampl sweep"
                n62 = local read "sine waves"() -> (w231:cluster{"freq":dbl, "ampl":dbl, "cycles":dbl}[])
                n63 = for {
                  tunnel: w231 -> [w246] mode=indexing
                  tunnel: [w245] -> w230 mode=indexing
                  tunnel: [w244] -> w229 mode=indexing
                  n64 = Unbundle By Name(w246) -> ("freq"=w245:dbl, "ampl"=w244:dbl)
                }
                n65 = case shown="0, Default" w226 {
                  tunnel: w230 -> [_ w240]
                  tunnel: w229 -> [w235 _]
                  tunnel: 1e-06 -> [w233 w239]
                  tunnel: [w232 w238] -> w227
                  frame 0, Default {
                    # "freq sweep"
                    n66 = Array Max & Min(array=w235) -> (max value=w236:dbl, min value=w237:dbl)  [unwired: 2 out]
                    n67 = Subtract(x=w236, y=w237) -> (x-y=w234:dbl)
                    n68 = Less?(x=w234, y=w233) -> (x < y?=w232:bool)
                  }
                  frame 2 {
                    # "ampl sweep"
                    n69 = Array Max & Min(array=w240) -> (max value=w242:dbl, min value=w243:dbl)  [unwired: 2 out]
                    n70 = Subtract(x=w242, y=w243) -> (x-y=w241:dbl)
                    n71 = Less?(x=w241, y=w239) -> (x < y?=w238:bool)
                  }
                }
                "use level" <- w227
              }
              frame Default {
              }
            }
          }
          frame #2 {
            n72 = local read "use level"() -> (w257:bool)
            n73 = Equal?(x="sweep type", y=5) -> (x = y?=w259:bool)
            n74 = Equal To 0?(x="sweep type") -> (x = 0?=w258:bool)
            n75 = Or(x=w258, y=w259) -> (x .or. y?=w255:bool)
            n76 = And(x=w255, y=w257) -> (x .and. y?=w253:bool)
            n77 = Compound Arithmetic op=AND(invert w255, w257) -> (w254:bool)
            n78 = local read "EQ Curve"() -> (w249:T3)
            n79 = Bundle(w254, w253, "ApplyEQ"=w251) -> (w250:cluster{bool, bool, "ApplyEQ":bool})  [unwired: 1 out]
            n80 = case shown="Default" "sweep type" {
              selector: "sweep type" -> [w272 _ _ _ _ _]
              tunnel: "Channel Out" -> [_ _ _ w379 _ _]
              tunnel: "Level Out" -> [w277 w357 w372 w381 w401 w425]
              tunnel: [w270 w351 w362 sgl[] [] w399 w428] -> w260
              tunnel: [w275 TRUE ("Verdict") w367 w376 TRUE ("Verdict") TRUE ("Verdict")] -> w265
              tunnel: w264 -> [w269 _ w366 _ w397 _]
              tunnel: w251 -> [w274 _ _ _ _ _]
              tunnel: [w273 _ _ _ _ _] -> w263
              tunnel: w262 -> [_ _ _ _ _ w427]
              tunnel: w261 -> [w271 _ _ _ _ _]
              tunnel: w250 -> [_ w350 w361 _ w391 w414]
              tunnel: w249 -> [w267 w349 w360 _ w392 w415]
              frame Default {
                # "???????????"
                # "freq stepped or log ampl sweep or two tone"
                n81 = case shown="False" FALSE {
                  tunnel: [sgl 0.0 w297] -> w281
                  tunnel: [sgl 0.0 w301] -> w280
                  tunnel: [w282 w300] -> w279
                  tunnel: [w282 w299] -> w278
                  tunnel: [w282 w298] -> w268
                  tunnel: "sine waves" -> [_ w289]
                  frame False {
                    w282 = FALSE
                  }
                  frame True {
                    n82 = Array Size(array="Eq") -> (size(s)=w293:i32)
                    "EQ Steps" <- w293
                    n83 = for {
                      tunnel: w289 -> [w303] mode=indexing
                      tunnel: [w302] -> w288 mode=indexing
                      n84 = Unbundle By Name(w303) -> ("freq"=w302:dbl)
                    }
                    n85 = Decrement(x=w293) -> (x-1=w292:i32)
                    n86 = Index Array(array="Eq", index=w292) -> (element=w296:cluster{"Hz":sgl, "dB":sgl, "Deg":sgl})
                    n87 = Index Array(array="Eq", index=0) -> (element=w295:cluster{"Hz":sgl, "dB":sgl, "Deg":sgl})
                    n88 = Array Max & Min(array=w288) -> (max value=w287:dbl, min value=w286:dbl)  [unwired: 2 out]
                    n89 = Unbundle By Name(w295) -> ("Hz"=w290:sgl)
                    n90 = Unbundle By Name(w296) -> ("Hz"=w291:sgl)
                    n91 = Max & Min(x=w290, y=w291) -> (max(x,y)=w297:sgl, min(x,y)=w301:sgl)
                    n92 = Greater?(x=w287, y=w297) -> (0:w299:bool)
                    n93 = Less?(x=w286, y=w301) -> (x < y?=w300:bool)
                    n94 = Or(x=w300, y=w299) -> (x .or. y?=w298:bool)
                  }
                }
                n95 = case shown="False" w268 {
                  tunnel: w278 -> [_ w334]
                  tunnel: w279 -> [_ w333]
                  tunnel: w280 -> [_ w332]
                  tunnel: w281 -> [_ w331]
                  tunnel: w274 -> [w320 _]
                  tunnel: [w323 sgl[] []] -> w270
                  tunnel: w272 -> [w318 _]
                  tunnel: "sine waves" -> [w315 _]
                  tunnel: w277 -> [w319 _]
                  tunnel: [TRUE ("Verdict") FALSE ("Verdict")] -> w275
                  tunnel: w269 -> [w314 _]
                  tunnel: [w312 _] -> w273
                  tunnel: w271 -> [w309 _]
                  tunnel: w267 -> [w308 _]
                  frame False {
                    # "Not use"
                    n96 = local read "use level"() -> (w307:bool)
                    n97 = Equal?(x=w318, y=5) -> (x = y?=w327:bool)
                    n98 = Equal To 0?(x=w318) -> (x = 0?=w326:bool)
                    n99 = Or(x=w326, y=w327) -> (x .or. y?=w324:bool)
                    n100 = And(x=w324, y=w307) -> (x .and. y?=w321:bool)
                    n101 = Compound Arithmetic op=AND(invert w324, w307) -> (w322:bool)
                    n102 = Bundle("sweep type"=w318, "Sampling Rate"="Sampling Rate", "Frequency"="Frequency", "Start Amplitude"="Start Amplitude", "Level Out"=w319) -> (w317:T26)  [unwired: 1 out]
                    n103 = Bundle(w322, w321, "ApplyEQ"=w320) -> (w316:cluster{bool, bool, "ApplyEQ":bool})  [unwired: 1 out]
                    n104 = local read "FAPS"() -> (w310:T7)
                    n105 = call "CRYFreq or Log Amp Sweep.vi"("Output Flag"=w316, "Stimulus Para"=w314, "end"=w309, "FAPS in"=w310, "Master sine waves"=w315, "EQ Curve"=w308, "Param1"=w317) -> ("FAPS out"=w313:T7, "Stimulus out"=w311:sgl[], "Diff Frequency"=w312:dbl)  [unwired: 2 in]
                    n106 = local write "FAPS"(w313) -> ()
                    n107 = To Single Precision Float(number=w311) -> (single precision float=w323:sgl[])
                  }
                  frame True {
                    n108 = case shown="True" w333 {
                      tunnel: w332 -> [_ w338]
                      frame False {
                      }
                      frame True {
                        n109 = call "CRYGet Error Message.vi"("Error No"=5, "Kind"="Stimulus") -> ("Message"=w335:string, "Window Title"=w336:string)  [unwired: 4 in, 4 out]
                        n110 = Format Into String(format string=w335, w338) -> (resulting string=w337:string)  [unwired: 2 in, 1 out]
                        n111 = call "CRYMessage Dialog.vi"("Window Title"=w336, "Message Content"=w337) -> ()  [unwired: 8 in, 2 out]
                      }
                    }
                    n112 = case shown="True" w334 {
                      tunnel: w331 -> [_ w344]
                      frame False {
                      }
                      frame True {
                        n113 = call "CRYGet Error Message.vi"("Error No"=6, "Kind"="Stimulus") -> ("Message"=w341:string, "Window Title"=w342:string)  [unwired: 4 in, 4 out]
                        n114 = Format Into String(format string=w341, w344) -> (resulting string=w343:string)  [unwired: 2 in, 1 out]
                        n115 = call "CRYMessage Dialog.vi"("Window Title"=w342, "Message Content"=w343) -> ()  [unwired: 8 in, 2 out]
                      }
                    }
                  }
                }
              }
              frame 1 {
                # "???? there is increase case.  if sweep time is large. ????"
                # "freq log sweep"
                n116 = local read "Start Frequency"() -> (w355:dbl)
                n117 = local read "Stop Frequency"() -> (w354:dbl)
                n118 = local read "Sampling Rate"() -> (w356:dbl)
                n119 = call "CRYFreq Log Sweep.vi"("Output Flag"=w350, "Amplitude"=w357, "EQ Curve"=w349, "Sweep time"="Sweep Time", "Fstop"=w354, "Fstart"=w355, "Fs"=w356) -> ("EQ Amplitude Rate"=→"EQ Amplitude Rate":dbl, "TSR params"=w358:T6, "Analysis"=w352:dbl[], "Sweep"=w353:dbl[])  [unwired: 1 in]
                n120 = local write "Analysis Value"(w352) -> ()
                n121 = local write "TSR params"(w358) -> ()
                n122 = To Single Precision Float(number=w353) -> (single precision float=w351:sgl[])
              }
              frame 3 {
                # "selected Wave file channel."
                # "wav file"
                n123 = Unbundle By Name(w366) -> ("Tone type6"=w365:u16)
                n124 = call "CRYStimulus Wave.vi"("EQ Curve"=w360, "Output Flag"=w361, "Max level"="max level", "Level Out"=w372, "wav path"="wav path") -> ("Verdict"=w367:bool, "Stop Frequency"=w368:dbl, "Start Frequency"=w369:dbl, "Sampling Rate"=w370:dbl, "R"=w364:sgl[], "L"=w363:sgl[])  [unwired: 1 out]
                n125 = local write "Sampling Rate"(w370) -> ()
                n126 = local write "Start Frequency"(w369) -> ()
                n127 = local write "Stop Frequency"(w368) -> ()
                n128 = case shown="0, Default" w365 {
                  tunnel: w364 -> [_ w375]
                  tunnel: w363 -> [w374 _]
                  tunnel: [w374 w375] -> w362
                  frame 0, Default {
                  }
                  frame 1 {
                  }
                }
              }
              frame 4 {
                # "dc volts"
                n129 = Decrement(x=w379) -> (x-1=w380:i32)
                n130 = call "CRYDc volts out visa.vi"("Volts"=w381, "COM port (0=COM1, etc.)"=w380) -> ("error"=w377:bool)  [unwired: 9 out]
                n131 = case shown="True" w377 {
                  tunnel: w379 -> [_ w385]
                  frame False {
                  }
                  frame True {
                    n132 = call "CRYGet Error Message.vi"("Error No"=8, "Kind"="Stimulus") -> ("Message"=w384:string, "Window Title"=w382:string)  [unwired: 4 in, 4 out]
                    n133 = Format Into String(format string=w384, w385) -> (resulting string=w383:string)  [unwired: 2 in, 1 out]
                    n134 = call "CRYMessage Dialog.vi"("Window Title"=w382, "Message Content"=w383) -> ()  [unwired: 8 in, 2 out]
                  }
                }
                n135 = Not(x=w377) -> (.not. x?=w376:bool)
              }
              frame 6 {
                n136 = Unbundle By Name(w397) -> ("Tone type6"=w398:u16)
                n137 = local read "Sweep Time"() -> (w390:dbl)
                n138 = case shown="1" w398 {
                  tunnel: [w405 w406] -> w402
                  frame 0, Default {
                    w405 = u16 1 items=["White Noise", "Pink Noise"] ("Noise type")
                  }
                  frame 1 {
                    w406 = u16 0 items=["White Noise", "Pink Noise"] ("Noise type")
                  }
                }
                n139 = local read "Sampling Rate"() -> (w403:dbl)
                n140 = local read "max level"() -> (w394:dbl)
                n141 = local read "Y dB ref"() -> (w395:dbl)
                n142 = local read "Unit"() -> (w393:u16)
                n143 = Bundle("Unit"=w393, "max level"=w394, "Y dB ref"=w395) -> (w396:T27)  [unwired: 1 in]
                n144 = call "CRYNoise White Pink.vi"("Fs"=w403, "Setting Infor"=w396, "EQ Curve"=w392, "Output Flag"=w391, "Min Frequency"="Start Frequency", "Max Frequency"="Stop Frequency", "Time(s)"=w390, "Amplitude"=w401, "Noise type"=w402) -> ("Noise"=w404:sgl[])  [unwired: 1 in, 5 out]
                n145 = To Single Precision Float(number=w404) -> (single precision float=w399:sgl[])
              }
              frame 7 {
                n146 = Unbundle By Name(w427) -> ("mltitone"=w426:T22)
                n147 = Unbundle By Name(w426) -> ("Freq Rounding"=w420:bool, "Rounding Val"=w419:dbl)
                n148 = local read "Sweep Time"() -> (w411:dbl)
                n149 = local read "max level"() -> (w417:dbl)
                n150 = local read "Y dB ref"() -> (w416:dbl)
                n151 = local read "Start Frequency"() -> (w410:dbl)
                n152 = local read "Stop Frequency"() -> (w409:dbl)
                n153 = local read "Sampling Rate"() -> (w412:dbl)
                n154 = local read "Unit"() -> (w418:u16)
                n155 = local read "Resolution"() -> (w408:u16)
                n156 = local read "Steps"() -> (w407:u32)
                n157 = Bundle("Start Frequency"=w410, "Stop Frequency"=w409, "Steps"=w407, "Sweep Time"=w411, "Level Out"=w425, "Level Out"=0.0, "Unit"=w418, "max level"=w417, "Y dB ref"=w416) -> (w423:T28)  [unwired: 1 in]
                n158 = local read "FAPS"() -> (w422:T7)
                n159 = call "CRYMultitone.vi"("Stimulus Infor"=w423, "EQ Curve"=w415, "Output Flag"=w414, "FAPS In"=w422, "Fs"=w412, "Resolution"=w408, "Freq Rounding"=w420, "Freq Rounding Value"=w419) -> ("tones"=w430:dbl[], "FAPS"=w421:T7, "EQ Amplitude Rate"=w413:dbl)  [unwired: 3 in, 2 out]
                n160 = local write "FAPS"(w421) -> ()
                n161 = local write "EQ Amplitude Rate"(w413) -> ()
                n162 = To Single Precision Float(number=w430) -> (single precision float=w428:sgl[])
              }
            }
          }
        }
        n163 = Build Array (concatenate)(w148, w146) -> (w147:sgl[])
        n164 = And(x=w143, y=w144) -> (x .and. y?=w145:bool)
      }
      n165 = call "CRYCheck String Array Equal.vi"("In Array"=w53) -> ("Equal"=w50:bool, "Name String"=w51:string)  [unwired: 9 out]
      n166 = flat-sequence {
        tunnel: w31 -> [w99]
        tunnel: w63 -> [w98]
        tunnel: w60 -> [w97]
        tunnel: w59 -> [w96]
        tunnel: [w95] -> w52
        tunnel: w51 -> [w94]
        tunnel: w50 -> [w92]
        tunnel: w32 -> [w78]
        tunnel: [w73] -> w13
        tunnel: [w76] -> w12
        tunnel: w9 -> [w75]
        frame #0 {
          w79 = T29 {"Stimulus Type"="", "Signal Type"="", "In/Out"=FALSE, "FAPS"=[], "Sampling Rate"=0.0, "Samples"=0, "Analysis Param"="", "Resolution"=0, "Steps"=0, "Analysis Value"=[], "Diff Freq"=0.0, "FStart"=0.0, "FStop"=0.0, "Calibration Param"="", "Anti Alias"=0.0, "Level Out1"=0.0, "Level Out2"=0.0, "EQ"=FALSE}  # unflattened test infor data
          n167 = local read "Sampling Rate"() -> (w73:dbl)
          n168 = local read "Calibration All Cluster"() -> (w83:T4)
          n169 = local read "Y unit"() -> (w76:string)
          n170 = local read "TSR params"() -> (w77:T6)
          n171 = local read "EQ Amplitude Rate"() -> (w74:dbl)
          n172 = local read "FAPS"() -> (w91:T7)
          n173 = Array Size(array=w99) -> (size(s)=w88:i32)
          n174 = local read "Start Frequency"() -> (w85:dbl)
          n175 = local read "Stop Frequency"() -> (w84:dbl)
          n176 = local read "Level Out"() -> (w80:dbl)
          n177 = Select(t=w91, s=w92, f=T7 [] ("FAPS")) -> (s? t:f=w90:T7)
          n178 = Flatten To String(anything=w77) -> (data string=w87:string)  [unwired: 1 in, 4 out]
          n179 = Flatten To String(anything=w83) -> (data string=w82:string)  [unwired: 1 in, 4 out]
          n180 = Bundle By Name(cluster=w79, "Stimulus Type"=w94, "Signal Type"=w96, "FAPS"=w90, "Sampling Rate"=w73, "Samples"=w88, "Analysis Param"=w87, "Resolution"=w98, "Steps"=w97, "Analysis Value"=dbl[] [], "Diff Freq"=w78, "In/Out"=FALSE, "FStart"=w85, "FStop"=w84, "Calibration Param"=w82, "Level Out1"=w80, "EQ"=w75, "Level Out2"=w74) -> (w93:T29)
          n181 = call "CRYFlatten Test Infor.vi"("Test Infor data"=w93) -> ("Fattened Data"=w95:string)  [unwired: 10 out]
        }
      }
      n182 = global read "CRYProject Run Control Global.vi" "RunState"() -> (w38:bool)
      n183 = Reciprocal(x=w13) -> (1/x=w48:dbl)
      n184 = Bundle By Name(cluster="Waveform Cluster", "X data"=w46, "Y data"=w46, "Waveform.dX"=w48, "Waveform.Y"=w31, "Name"=w15, "Plot Settings.Color"=u32 16514929, "Step No."=w26, "X unit"="s", "Y unit"=w12, "Test Info"=w52) -> (w45:T1)
      n185 = case shown="False" w38 {
        tunnel: ["Apply" ("sOption1") "Run" ("Type In")] -> w37
        tunnel: ["APPLY_CURVE" ("Type In") "RUN_CURVE" ("Type In")] -> w36
        frame False {
        }
        frame True {
        }
      }
      n186 = call "CRYCalc FSD.vi"("Max Level"=w18, "X"=w31) -> ("dBFSD(RMS)"=w21:dbl, "%FSD(RMS)"=w22:dbl)  [unwired: 6 in, 2 out]
      n187 = Build Array(w45) -> (w40:T1[])
      "Wave out" <- w40
      n188 = Index Array(array=w55, index=1) -> (element=w39:bool)
      n189 = call "CRYUnflatten Results.vi"() -> ("Result"=w65:T9)  [unwired: 1 in, 10 out]
      n190 = Bundle By Name(cluster=w65, "Verdict"=w66) -> (w69:T9)
      n191 = Build Array(w69) -> (→"Results out":T9[])
      n192 = Select(t="Overwrite" ("Y unit"), s=w39, f="Repeat") -> (s? t:f=w41:string)
      n193 = Bundle By Name(cluster=cluster{"x":dbl, "y":dbl, "z":dbl} {"x"=0.0, "y"=0.0, "z"=0.0}, "x"=w22, "y"=w21) -> (w24:cluster{"x":dbl, "y":dbl, "z":dbl})
      n194 = Build Array(w24) -> (w23:cluster{"x":dbl, "y":dbl, "z":dbl}[])
      n195 = call <vilib>:"Space Constant.vi"() -> ("String"=w16:string)
      n196 = Concatenate Strings("Max FSD Out" ("Name"), w16, w15) -> (w14:string)
      n197 = Bundle By Name(cluster=w30, "Name"=w14, "Curve"=w23, "Step No."=w26, "single val"=w10, "X unit"="%FSD", "Y unit"="dBFSD", "display X"=w10, "display Y"=w10, "display Z"=FALSE) -> (w29:T3)
      n198 = Build Array(w29) -> (w20:T3[])
      "Data out" <- w20
      n199 = case shown="True" w39 {
        tunnel: w36 -> [w109 _]
        tunnel: w40 -> [w108 w111]
        tunnel: [w107 w111] -> w33
        tunnel: w54 -> [w106 _]
        tunnel: w20 -> [w105 w110]
        tunnel: [w104 w110] -> w19
        frame False {
          n200 = call "CRYPrefix Curve Name.vi"("Type In"=w109, "Values In"=w105, "Waves In"=w108, "Repeat State Array In"=w106) -> ("Values Out"=w104:T10, "Waves Out"=w107:T30)  [unwired: 8 in, 2 out]
        }
        frame True {
        }
      }
      n201 = call "CRYInsert Socket.vi"("sOption2"=w41, "Step No."=w26, "sOption1"=w37, "Waves"=w33, "Values"=w19) -> ("Inserted Names Out"=→"Inserted Names Out":string[])  [unwired: 6 in]
    }
  }
